vi "Write 1D String.vi"(8 "error in":errorcluster, 9 "Write/Read Cell":T1={"Cell Range"="", "Data 2D"=[], "Select Sheet"="", "1 Data"="", "Data 1D"=[], "Font col"=0, "Bold"=TRUE, "Font Size"=18, "Inside lines"=FALSE}, 11 "Work Sheet 2":refnum<k7>) -> (0 "error out":errorcluster, 3 "Work Sheet":refnum<k7>)   [LabVIEW 2017]
uses:
  controls/read.write.ctl
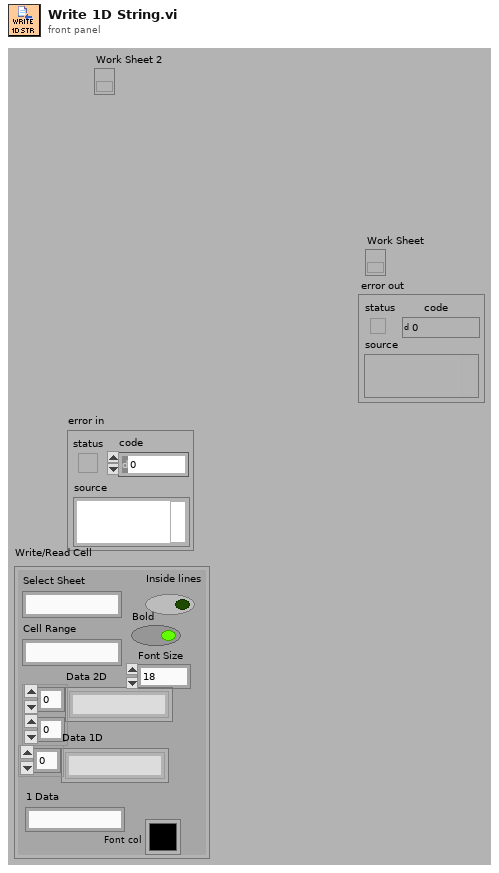
[diagram p1: front panel]
types:
  T1 = typedef "read.write.ctl" = cluster{"Cell Range":string, "Data 2D":string[][], "Select Sheet":string, "1 Data":string, "Data 1D":string[], "Font col":u32, "Bold":bool, "Font Size":i32, "Inside lines":bool}
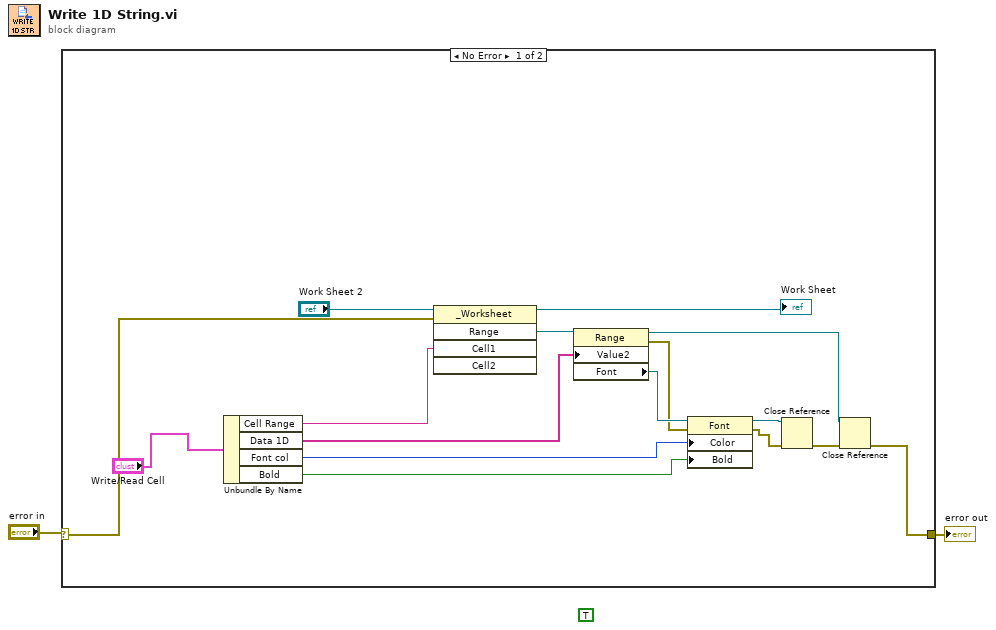
[diagram p0: block diagram]
diagram:
  (unwired) TRUE
  n1 = case shown="No Error" "error in" {
    selector: "error in" -> [w17 w19]
    tunnel: [w6 w19] -> w1
    frame No Error {
      n2 = Unbundle By Name("Write/Read Cell") -> ("Cell Range"=w3:string, "Data 1D"=w15:string[], "Font col"=w12:u32, "Bold"=w4:bool)
      n3 = invoke class="_Worksheet" method="Range"(reference="Work Sheet 2", error in=w17, "Cell1"=w3) -> (reference out=→"Work Sheet":refnum<k7>, "Range"=w18:refnum<k7>)  [unwired: 2 in, 3 out]
      n4 = property class="Range"(reference=w18, "Value2"=w15) -> (reference out=w8:refnum<k7>, error out=w9:errorcluster, "Font"=w13:refnum<k7>)  [unwired: 1 in]
      n5 = property class="Font"(reference=w13, error in=w9, "Color"=w12, "Bold"=w4) -> (reference out=w11:refnum<k7>, error out=w10:errorcluster)
      n6 = Close Reference(reference=w11, error in (no error)=w10) -> (error out=w7:errorcluster)
      n7 = Close Reference(reference=w8, error in (no error)=w7) -> (error out=w6:errorcluster)
    }
    frame Error {
    }
  }
  "error out" <- w1
